vi "MLS ident.vi"() -> ()   [LabVIEW 2015]
uses:
  <vilib>/Platform/TimedLoop/XDataNode/timing_clust.ctl
  <vilib>/Platform/TimedLoop/XDataNode/nitl_modes.ctl
  <vilib>/Platform/TimedLoop/XDataNode/wakeup.ctl
  <vilib>/FPGAPlugInAG/myRIO-1900/niLvFpga_Open_myRIO-1900.vi
  <vilib>/rvi/interface/common/dynamic/niFpgaDynamicAddResources.vi
  <vilib>/Utility/file.llb/Write Delimited Spreadsheet (I64).vi
  <vilib>/Utility/file.llb/Write Delimited Spreadsheet (DBL).vi
  <vilib>/Utility/error.llb/Error Cluster From Error Code.vi
  <vilib>/rvi/errors/niLvFpgaAdjustHostInterfaceError.vi
  <vilib>/FPGAPlugInAG/Dynamic/niLvFpga_Close_Dynamic.vi
  <vilib>/rvi/interface/nirviOpenFPGA/nirviOpenFPGA.xnode
  FPGA Bitfiles/ACC20115_FPGATarget_CurrentControlle_W-6n2rsGK8k.lvbitx
  Misc/Current Controller.vi
  <vilib>/Platform/TimedLoop/XDataNode/XDataNode.xnode
  <vilib>/rvi/interface/nirviReadWriteControl/nirviReadWriteControl.xnode
  <vilib>/rvi/interface/nirviCloseFPGA/nirviCloseFPGA.xnode
  <vilib>/Analysis/NI_AALBase.lvlib
  <vilib>/rvi/interface/Simulation/niFpgaSimulationCallBeginRW.vi
  NiFpgaLv.dll
  <vilib>/Platform/TimedLoop/XDataNode/XDNodeRunTimeDep.lvlib
panel:
  out "error out":errorcluster
  in  "Stop":bool
  in  "Tab Control":enum32{"Monitor"}(tab)
  out "MLS":dbl[](graph)
  out "Sensor":dbl(graph)
  out "FPGA Status":bool
  out "Uniform White Noise":dbl[](graph)
  in  "MLS Samples":i64(slide)=1 scale=0.0..30.0
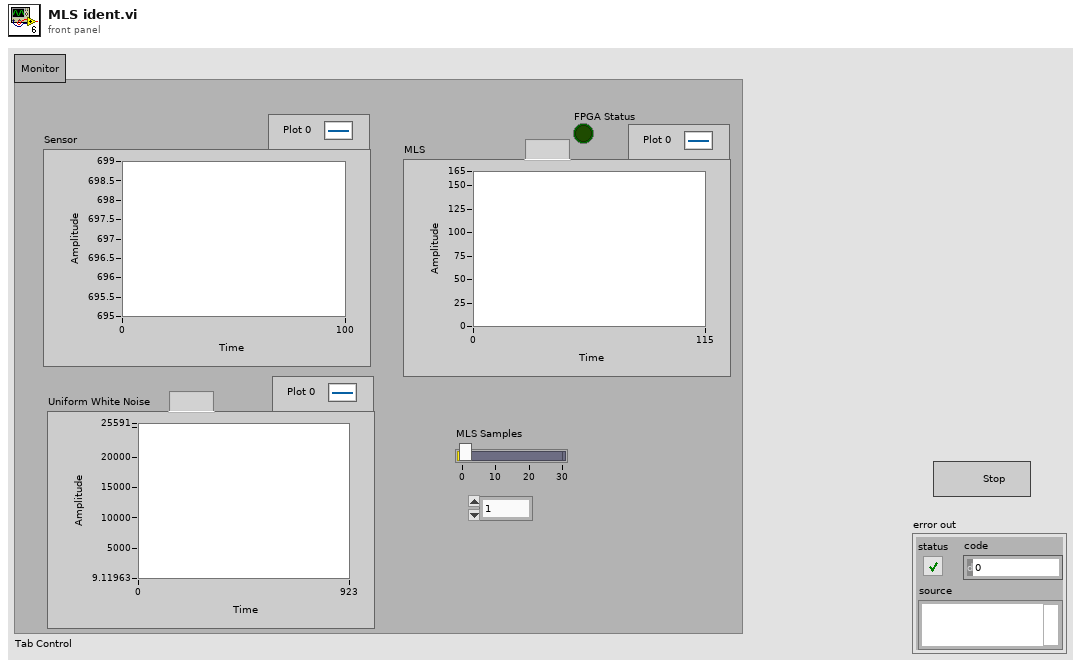
[diagram p1: front panel]
types:
  T1 = typedef "XDNodeRunTimeDep.lvlib/timing_clust.ctl" = cluster{"Expected End [f-1]":u64, "Actual End [f-1]":u64, "Finished Late? [f-1]":bool, "Expected End [i-1]":u64, "Actual End [i-1]":u64, "Finished Late? [i-1]":bool, "Expected Start [i]":u64, "Actual Start [i]":u64, "Expected Start [f]":u64, "Actual Start [f]":u64, "Source Name":string, "Structure Name":string, "Period":i64, "Deadline":i64, "Offset":i64, "Start":i64, "Priority":i32, "Timeout":i32, "Mode":T2, "Wakeup Reason":T3, "Error":errorcluster, "Source Type":string, "Secondary Source Type":string, "Global End Time":u64, "Global Start Time":u64, "Frame Duration":u64, "Iteration Duration":u64, "Assigned CPU":i32, "I/O Scan Engine Mode":u32}
  T2 = typedef "XDNodeRunTimeDep.lvlib/nitl_modes.ctl" = enum32{"No Change", "Process missed periods, maintain original phase", "Discard missed periods, maintain original phase", "Process missed periods, ignore original phase", "Discard missed periods, ignore original phase"}
  T3 = typedef "XDNodeRunTimeDep.lvlib/wakeup.ctl" = enum32{"Normal", "Aborted", "Asynchronous wakeup", "Timing source error", "Timed loop error", "Timeout"}
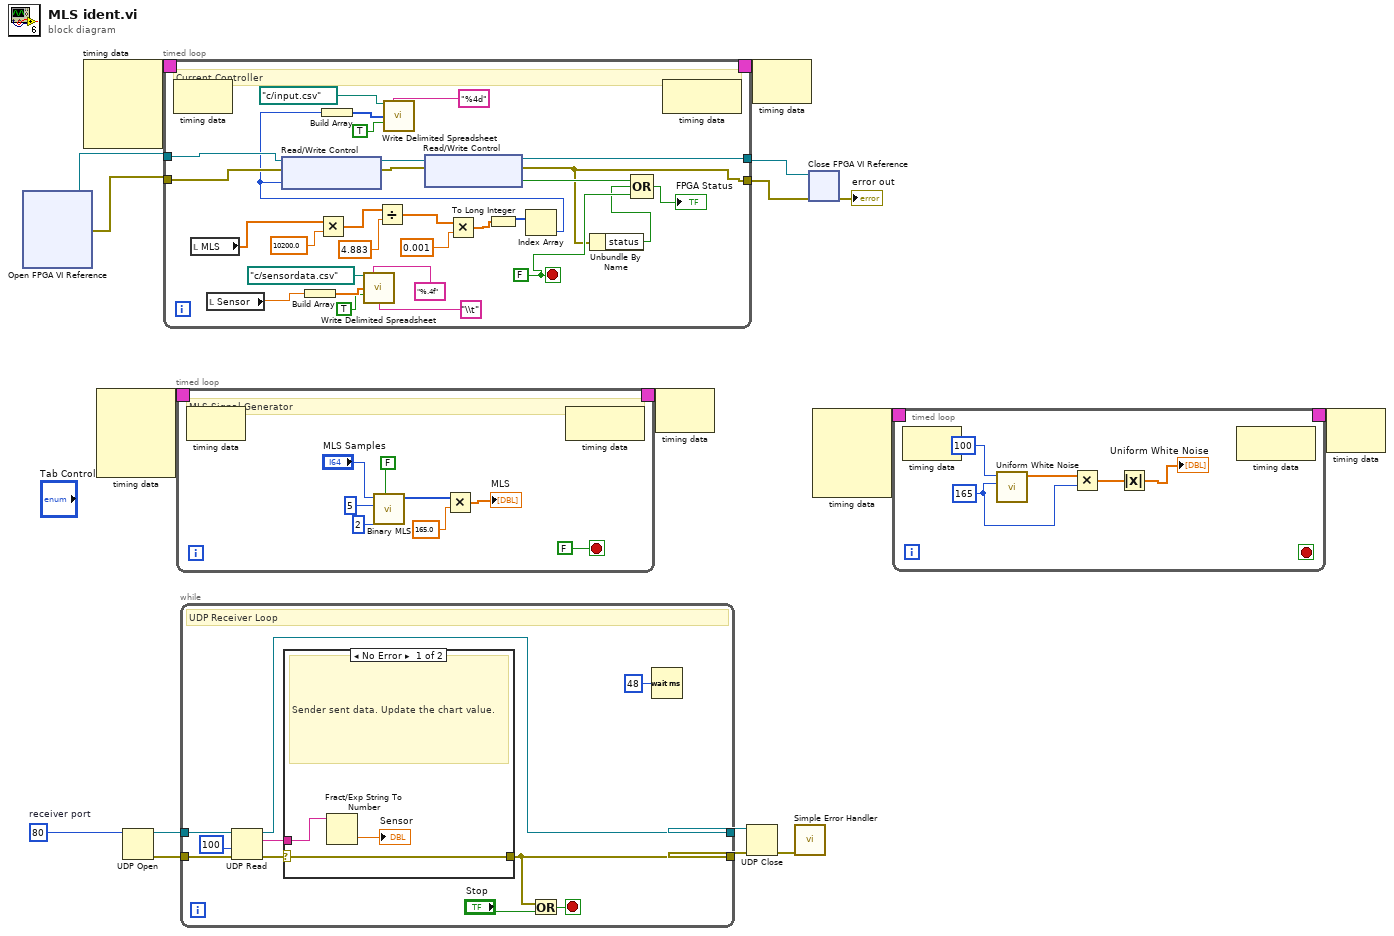
[diagram p0: block diagram]
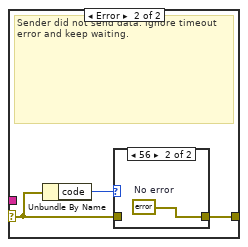
[diagram p2: hidden frame]
diagram:
  w8 = u16 80  # receiver port
  n1 = xnode "Open FPGA VI Reference"() -> ("FPGA VI Reference Out"=w17:refnum<k20>, "error out"=w16:errorcluster)  [unwired: 2 in]
  n2 = node-c288() -> (w2:T1)  [unwired: 4 in]
  n3 = node-c288() -> (w6:T1)  [unwired: 4 in]
  n4 = UDP Open(11:w8) -> (port=w9:refnum<k16>, 0:w10:errorcluster)  [unwired: 4 in, 1 out]
  n5 = timed-loop {
    tunnel: w17 -> [w46]
    tunnel: w16 -> [w45]
    tunnel: [w35] -> w15
    tunnel: [w31] -> w14
    timing: w2 -> [_]
    timing-out: [_] -> w1
    stop <- w34 stop-if-true
    w34 = FALSE
    # "Current Controller"
    n6 = node-c288() -> ()  [unwired: 1 in, 1 out]
    n7 = local read "MLS"() -> (w40:dbl[])
    n8 = local read "Sensor"() -> (w22:dbl)
    n9 = Build Array(w22) -> (w23:dbl[])
    n10 = Multiply(x=w40, y=10200.0) -> (x*y=w41:dbl[])
    n11 = call-poly <vilib>:"Write Delimited Spreadsheet.vi"("file path (dialog if empty)"=path "c:/sensordata.csv", "format (%.3f)"="%.4f", "1D data"=w23, "append to file? (F)"=TRUE, "delimiter (\\t)"="\\t" ("delimiter (\\t)")) -> ()  [unwired: 9 in, 2 out]
    n12 = Divide(x=w41, y=4.883) -> (x/y=w43:dbl[])
    n13 = Multiply(x=w43, y=0.001) -> (x*y=w39:dbl[])
    n14 = To Long Integer(number=w39) -> (32bit integer=w29:i32[])
    n15 = Index Array(array=w29) -> (element=w28:i32)  [unwired: 1 in]
    n16 = xnode "Read/Write Control"("FPGA VI Reference In"=w46, "error in"=w45, "DAC Inlet Valve"=w28) -> ("FPGA VI Reference Out"=w37:refnum<k20>, "error out"=w36:errorcluster)
    n17 = Build Array(w28) -> (w27:i32[])
    n18 = call-poly <vilib>:"Write Delimited Spreadsheet.vi"("file path (dialog if empty)"=path "c:/input.csv", "format (%d)"="%4d", "1D data"=w27, "append to file? (F)"=TRUE) -> ()  [unwired: 10 in, 2 out]
    n19 = xnode "Read/Write Control"("FPGA VI Reference In"=w37, "error in"=w36) -> ("FPGA VI Reference Out"=w35:refnum<k20>, "error out"=w31:errorcluster, "Inlet Overflow?"=w32:bool)
    n20 = Unbundle By Name(w31) -> ("status"=w33:bool)
    n21 = Compound Arithmetic op=OR(w32, w33, w34) -> (→"FPGA Status":bool)
    n22 = node-c288() -> ()  [unwired: 1 in, 1 out]
  }
  n23 = timed-loop {
    timing: w6 -> [_]
    timing-out: [_] -> w5
    stop <- FALSE stop-if-true
    # "MLS Signal Generator"
    n24 = node-c288() -> ()  [unwired: 1 in, 1 out]
    n25 = call <vilib>:"Binary MLS.vi"("initialize?"=FALSE, "seed"=i64 2, "polynomial order"=5, "samples"="MLS Samples") -> ("mls sequence"=w54:u8[])  [unwired: 6 in, 1 out]
    n26 = Multiply(x=w54, y=165.0 ("amplitude")) -> (x*y=→"MLS":dbl[])
    n27 = node-c288() -> ()  [unwired: 1 in, 1 out]
  }
  n28 = while {
    tunnel: w9 -> [w68]
    tunnel: [w60] -> w13
    tunnel: w10 -> [w65]
    tunnel: [w61] -> w11
    stop <- w66 stop-if-true
    # "UDP Receiver Loop"
    n29 = UDP Read(connection ID=w68, timeout ms (25000)=100, 8:w65) -> (data out=w63:string, error out=w62:errorcluster, 3:w60:refnum<k16>)  [unwired: 3 out]
    n30 = case shown="No Error" w62 {
      selector: w62 -> [w69 w73]
      tunnel: w63 -> [w71 _]
      tunnel: [w69 w72] -> w61
      frame No Error {
        # "Sender sent data. Update the chart value."
        n31 = Fract/Exp String To Number(string=w71) -> (number=→"Sensor":dbl)  [unwired: 3 in, 1 out]
      }
      frame Error {
        # "Sender did not send data. Ignore timeout error and keep waiting."
        n32 = Unbundle By Name(w73) -> ("code"=w74:i32)
        n33 = case shown="56" w74 {
          tunnel: w73 -> [w75 _]
          tunnel: [w75 w76] -> w72
          frame Default {
          }
          frame 56 {
            w76 = errorcluster {"status"=FALSE, "code"=0, "source"=""}  # No error
          }
        }
      }
    }
    n34 = Or(x=w61, y="Stop") -> (x .or. y?=w66:bool)
    n35 = Wait (ms)(milliseconds to wait=u32 48) -> ()  [unwired: 1 out]
  }
  n36 = node-c288(w5) -> ()  [unwired: 1 out]
  n37 = UDP Close(connection ID=w13, 8:w11) -> (error out=w12:errorcluster)  [unwired: 1 out]
  n38 = node-c288(w1) -> ()  [unwired: 1 out]
  n39 = call <vilib>:"Simple Error Handler.vi"("error in (no error)"=w12) -> ()  [unwired: 1 in, 8 out]
  n40 = xnode "Close FPGA VI Reference"("FPGA VI Reference In"=w15, "error in"=w14) -> ("error out"=→"error out":errorcluster)
  n41 = node-c288() -> (w4:T1)  [unwired: 4 in]
  n42 = timed-loop {
    timing: w4 -> [_]
    timing-out: [_] -> w3
    stop <- _ stop-if-true
    w79 = 165 ("polynomial order")
    n43 = node-c288() -> ()  [unwired: 1 in, 1 out]
    n44 = call <vilib>:"Uniform White Noise.vi"("amplitude"=w79, "samples"=i64 100) -> ("uniform white noise"=w77:dbl[])  [unwired: 8 in, 1 out]
    n45 = Multiply(x=w77, y=w79) -> (x*y=w80:dbl[])
    n46 = Absolute Value(x=w80) -> (abs(x)=→"Uniform White Noise":dbl[])
    n47 = node-c288() -> ()  [unwired: 1 in, 1 out]
  }
  n48 = node-c288(w3) -> ()  [unwired: 1 out]
